vi "ClearIPS.vi"(3 "error in (no error)":errorcluster, 5 "address string (25)":string="25") -> (0 "error out":errorcluster)   [LabVIEW 2009]
uses:
  Instance           1 16Saved   ClearIPS .vi
panel:
  in  "IPS Commands":string="C0   Local & Locked\nC3  Remote & Unlocked\n\nA0  Hold\nA1  To Set Point\nA2 To Zero\n\nH0 Switch Heater OFF\nH1 Switch Heater ON\n\nJnn Set Target Field\n\nTnn Set Field Sweep Rate\n\n\n\n"
  out "Antwort":string="Device Clear"
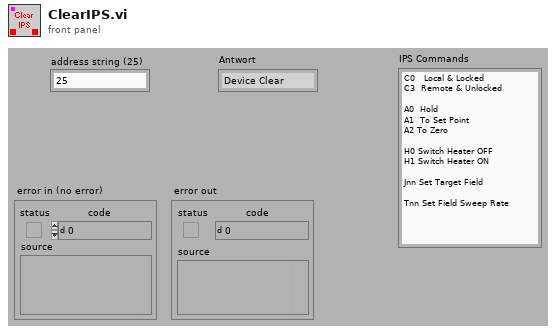
[diagram p1: front panel]
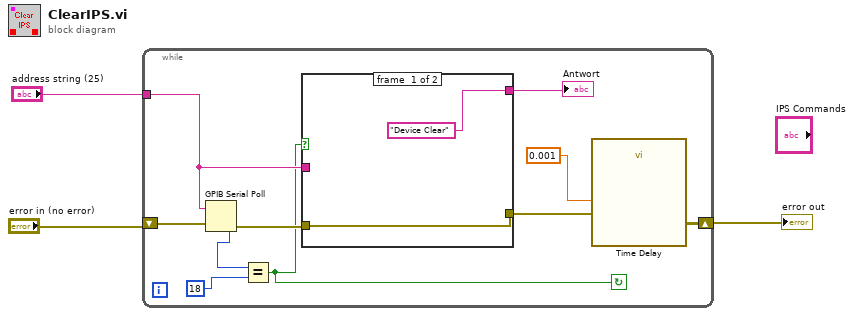
[diagram p0: block diagram]
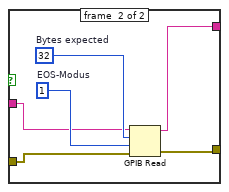
[diagram p2: hidden frame]
diagram:
  n1 = while {
    tunnel: "address string (25)" -> [w13]
    shift-right: [w5] -> w1
    shift-left: "error in (no error)" -> [w12]
    stop <- w8 continue-if-true
    n2 = GPIB Serial Poll(0:w13, 1:w12) -> (2:w10:i16, 4:w11:errorcluster)  [unwired: 1 out]
    n3 = Equal?(x=w10, y=18) -> (x = y?=w8:bool)
    n4 = case shown="True" w8 {
      tunnel: ["Device Clear" w19] -> w7
      tunnel: w13 -> [_ w18]
      tunnel: [w14 w17] -> w6
      tunnel: w11 -> [w14 w16]
      frame #0 {
      }
      frame #1 {
        w20 = 1  # EOS-Modus
        w21 = 32  # Bytes expected
        n5 = GPIB Read(0:w18, 1:w21, 2:w20, 3:w16) -> (5:w19:string, 7:w17:errorcluster)  [unwired: 1 in, 1 out]
      }
    }
    "Antwort" <- w7
    n6 = call "Time Delay"("error in (no error)"=w6, "Delay Time (s)"=0.001) -> ("error out"=w5:errorcluster)  [unwired: 9 in]
  }
  "error out" <- w1
